vi "DAQ Etch-A-Sketch.vi"() -> ()   [LabVIEW 2011]
uses:
  <vilib>/Platform/TimedLoop/XDataNode/timing_clust.ctl
  <vilib>/Platform/TimedLoop/XDataNode/nitl_modes.ctl
  <vilib>/Platform/TimedLoop/XDataNode/wakeup.ctl
  <vilib>/DAQmx/read.llb/DAQmx Read (Analog 1D DBL NChan 1Samp).vi
  <vilib>/DAQmx/create/channels.llb/DAQmx Create Channel (AI-Voltage-Basic).vi
  <vilib>/DAQmx/miscellaneous.llb/DAQmx Fill In Error Info.vi
  <vilib>/Platform/TimedLoop/XDataNode/XDataNode.xnode
  <vilib>/Platform/TimedLoop/XDataNode/XDNodeRunTimeDep.lvlib
panel:
  out "XY Graph":cluster{dbl[], dbl[]}(graph)
  out "collected voltages":dbl[][](array[numeric])
  out "loop iterator":i32
  out "data":dbl[](array[numeric]) format="%0.2f"
  out "error out":errorcluster
  in  "stop":bool
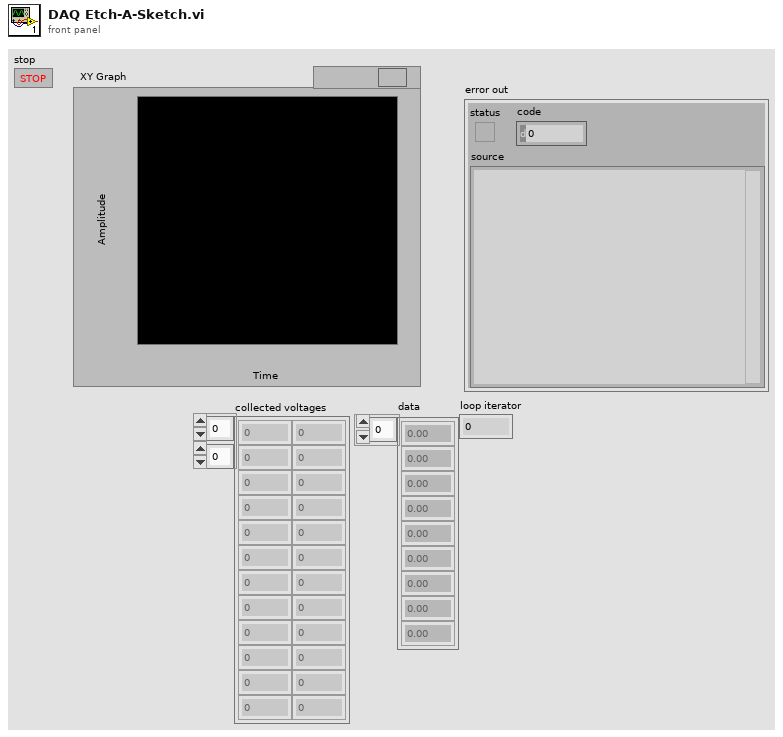
[diagram p1: front panel]
types:
  T1 = typedef "XDNodeRunTimeDep.lvlib/timing_clust.ctl" = cluster{"Expected End [f-1]":u64, "Actual End [f-1]":u64, "Finished Late? [f-1]":bool, "Expected End [i-1]":u64, "Actual End [i-1]":u64, "Finished Late? [i-1]":bool, "Expected Start [i]":u64, "Actual Start [i]":u64, "Expected Start [f]":u64, "Actual Start [f]":u64, "Source Name":string, "Structure Name":string, "Period":i64, "Deadline":i64, "Offset":i64, "Start":i64, "Priority":i32, "Timeout":i32, "Mode":T2, "Wakeup Reason":T3, "Error":errorcluster, "Source Type":string, "Secondary Source Type":string, "Global End Time":u64, "Global Start Time":u64, "Frame Duration":u64, "Iteration Duration":u64, "Assigned CPU":i32, "I/O Scan Engine Mode":u32}
  T2 = typedef "XDNodeRunTimeDep.lvlib/nitl_modes.ctl" = enum32{"No Change", "Process missed periods, maintain original phase", "Discard missed periods, maintain original phase", "Process missed periods, ignore original phase", "Discard missed periods, ignore original phase"}
  T3 = typedef "XDNodeRunTimeDep.lvlib/wakeup.ctl" = enum32{"Normal", "Aborted", "Asynchronous wakeup", "Timing source error", "Timed loop error", "Timeout"}
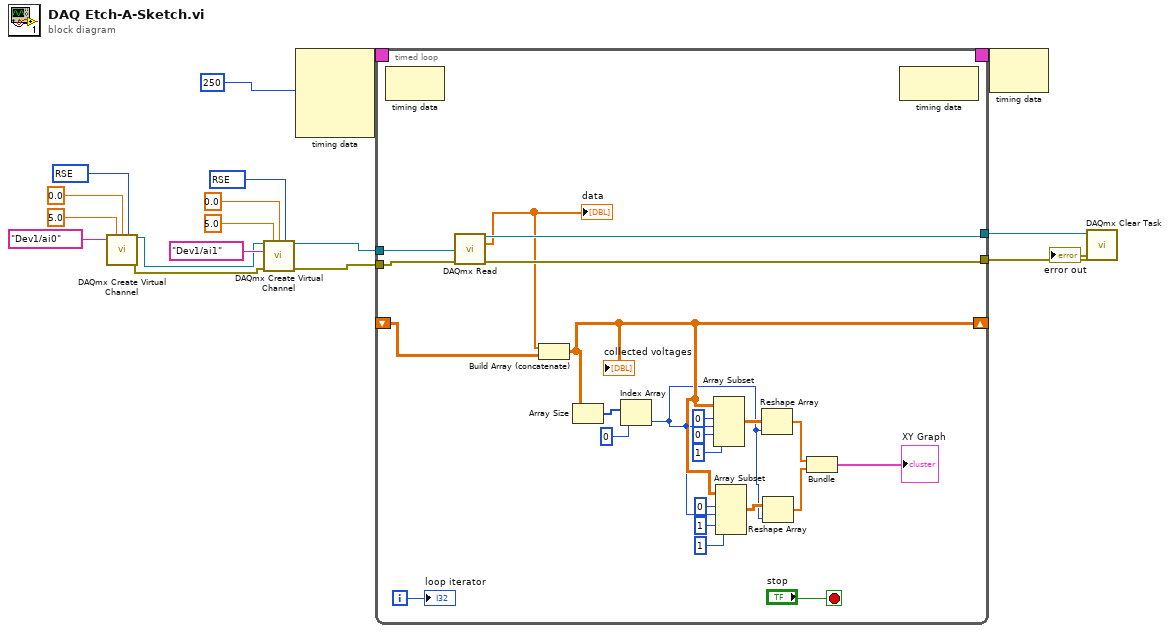
[diagram p0: block diagram]
diagram:
  w13 = 10083 items=["default"=-1, "RSE"=10083, "NRSE"=10078, "Differential"=10106, "Pseudodifferential"=12529] ("input terminal configuration")
  w16 = 10083 items=["default"=-1, "RSE"=10083, "NRSE"=10078, "Differential"=10106, "Pseudodifferential"=12529] ("input terminal configuration")
  n1 = call-poly <vilib>:"DAQmx Create Virtual Channel.vi"("maximum value"=5.0, "minimum value"=0.0, "input terminal configuration"=w16, "physical channels"=tag "Dev1/ai0") -> ("task out"=w10:refnum<k21>, "error out"=w9:errorcluster)  [unwired: 10 in]
  n2 = call-poly <vilib>:"DAQmx Create Virtual Channel.vi"("task in"=w10, "maximum value"=5.0, "minimum value"=0.0, "input terminal configuration"=w13, "physical channels"=tag "Dev1/ai1", "error in"=w9) -> ("task out"=w5:refnum<k21>, "error out"=w6:errorcluster)  [unwired: 8 in]
  n3 = node-c288(i64 250 ("Period")) -> (w4:T1)  [unwired: 3 in]
  n4 = timed-loop {
    timing: w4 -> [_]
    timing-out: [_] -> w3
    tunnel: [w41] -> w8
    tunnel: [w40] -> w7
    tunnel: w6 -> [w39]
    tunnel: w5 -> [w38]
    shift-right: [w31] -> _
    shift-left: _ -> [w35]
    i -> [w36]
    stop <- "stop" stop-if-true
    n5 = node-c288() -> ()  [unwired: 1 in, 1 out]
    n6 = call-poly <vilib>:"DAQmx Read.vi"("task/channels in"=w38, "error in"=w39) -> ("task out"=w41:refnum<k21>, "data"=w34:dbl[], "error out"=w40:errorcluster)  [unwired: 11 in]
    "data" <- w34
    n7 = Build Array (concatenate)(w34, w35) -> (w31:dbl[][])
    "collected voltages" <- w31
    n8 = Array Size(array=w31) -> (size(s)=w33:i32[])
    n9 = Index Array(array=w33, index=0) -> (element=w28:i32)
    n10 = Array Subset(array=w31, index (row)=0 ("index"), length (row)=w28, index (col)=0 ("index"), length (col)=1 ("length")) -> (w30:dbl[][])
    n11 = Array Subset(array=w31, index (row)=0 ("index"), length (row)=w28, index (col)=1 ("index"), length (col)=1 ("length")) -> (w29:dbl[][])
    n12 = Reshape Array(w30, w28) -> (w26:dbl[])
    n13 = Reshape Array(w29, w28) -> (w27:dbl[])
    n14 = Bundle(w26, w27) -> (→"XY Graph":cluster{dbl[], dbl[]})  [unwired: 1 in]
    n15 = node-c288() -> ()  [unwired: 1 in, 1 out]
    "loop iterator" <- w36
  }
  n16 = node-c288(w3) -> ()  [unwired: 1 out]
  n17 = call <vilib>:"DAQmx Clear Task.vi"("task in"=w8, "error in"=w7) -> ("error out"=→"error out":errorcluster)  [unwired: 13 in]
